vi "Excersie_5.vi"() -> ()   [LabVIEW 2013]
panel:
  in  "stop":bool
  out "Waveform Graph":dynamicdata(graph)
  in  "Square wave freq":dbl(slide) scale=0.0..10.0
  in  "Sin wave freq":dbl(slide) scale=0.0..10.0
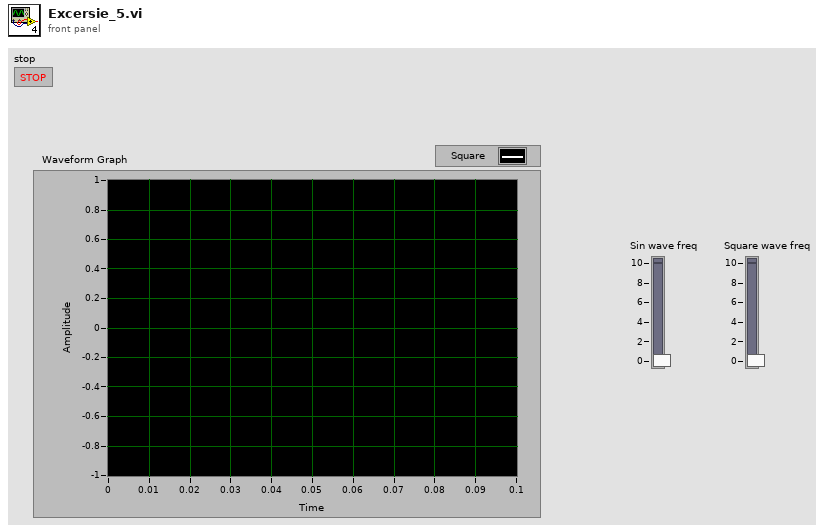
[diagram p1: front panel]
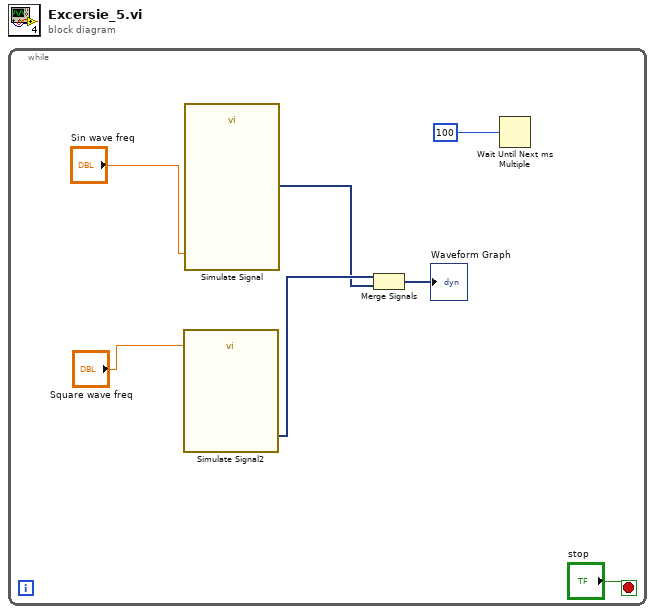
[diagram p0: block diagram]
diagram:
  n1 = while {
    stop <- "stop" stop-if-true
    n2 = call "Simulate Signal2"("Frequency"="Square wave freq") -> ("Square"=w3:dynamicdata)  [unwired: 13 in, 1 out]
    n3 = call "Simulate Signal"("Frequency"="Sin wave freq") -> ("Sine"=w1:dynamicdata)  [unwired: 13 in, 1 out]
    n4 = Merge Signals(w3, w1) -> (→"Waveform Graph":dynamicdata)
    n5 = Wait Until Next ms Multiple(millisecond multiple=u32 100) -> ()  [unwired: 1 out]
  }
